vi "laplace_transform.vi"() -> ()   [LabVIEW 2020]
uses:
  <vilib>/Analysis/2dsp.llb/Real FFT.vi
  <vilib>/express/express analysis/Spectral/Block/exnSpectralBlock spectral measurements power poly.vi
  <vilib>/express/express analysis/Spectral/Block/exnSpectralBlock spectral measurements power WFM.vi
  <vilib>/express/express analysis/Spectral/Block/exnSpectralBlock spectral measurements power DDT.vi
  <vilib>/express/express analysis/Spectral/XNode/ExpressSpectralMeasurementsBlockNode.xnode
  <vilib>/Analysis/NI_AALPro.lvlib
  <vilib>/gmath/NI_Gmath.lvlib
panel:
  in  "end":dbl format="%.2f"
  out "Laplace Transform":dbl[](graph)
  out "Filtered Spectral Measurement":dynamicdata(graph)
  out "Spectral Measurement":cluster{"f0":dbl, "df":dbl, "magnitude":dbl[]}(graph)
  in  "shift?":bool
  in  "FFT size":i32=-1
  out "Fast Fourier Transform Graph":dbl[](graph)
  out "Amplitude vs Time (Chart)":waveform(dbl)(graph)
  out "Amplitude vs Time (Graph)":waveform(dbl)(graph)
  in  "path":path
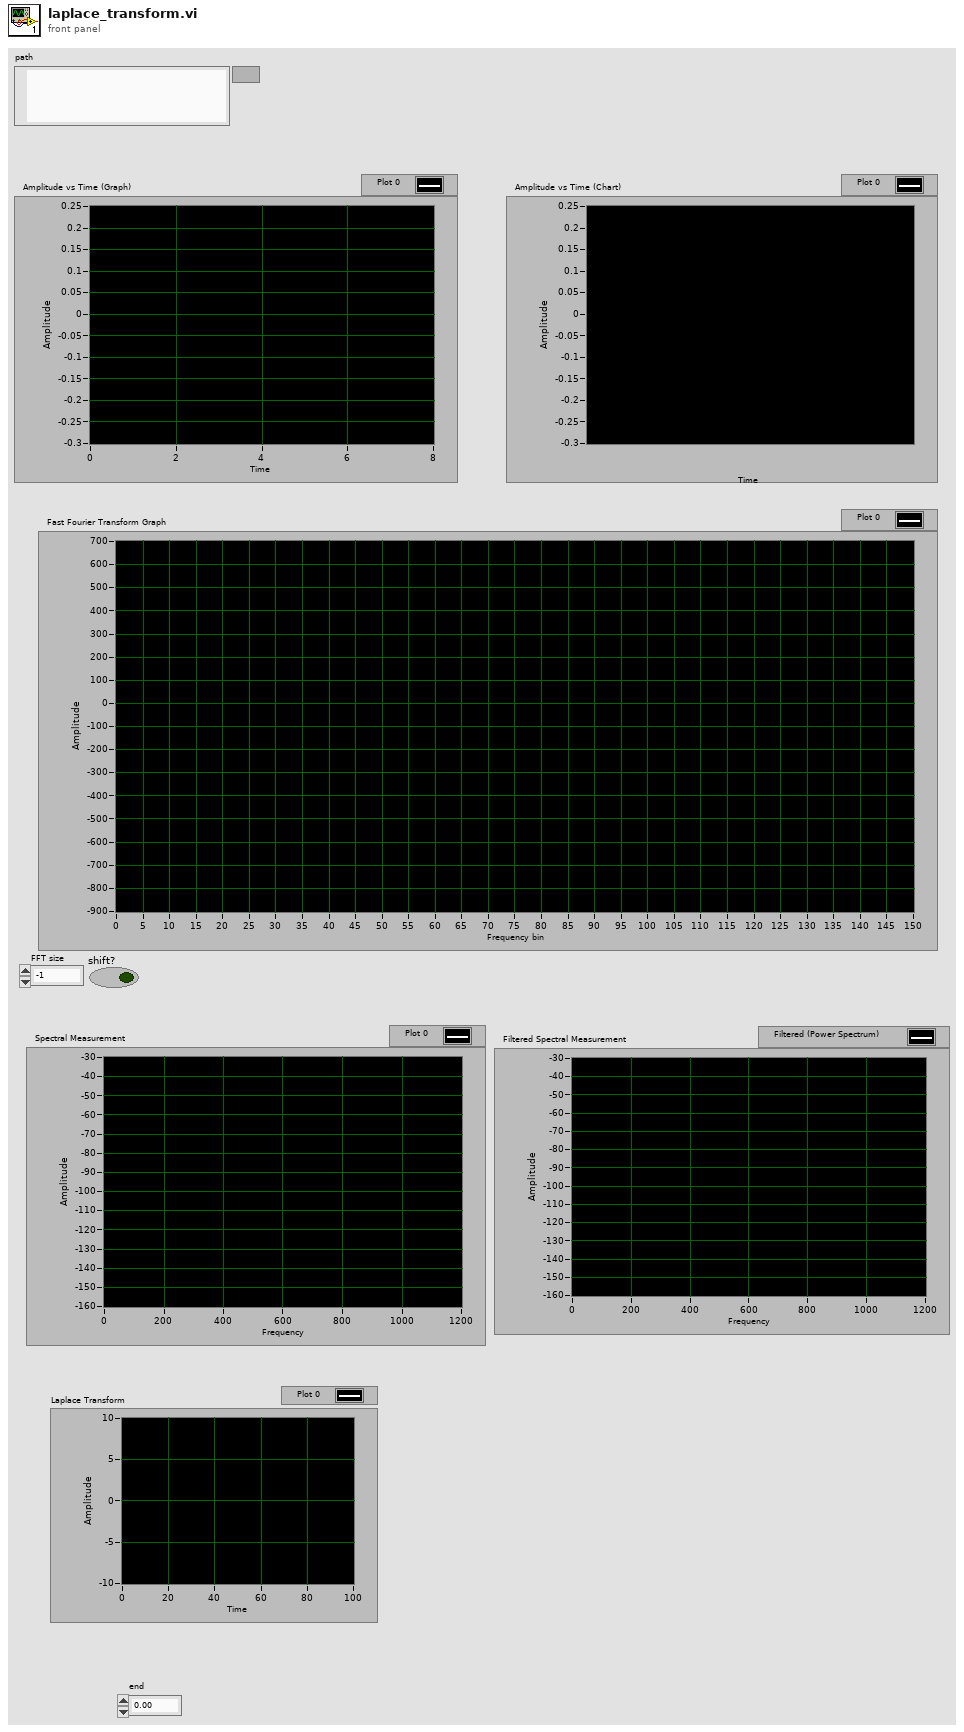
[diagram p1: front panel]
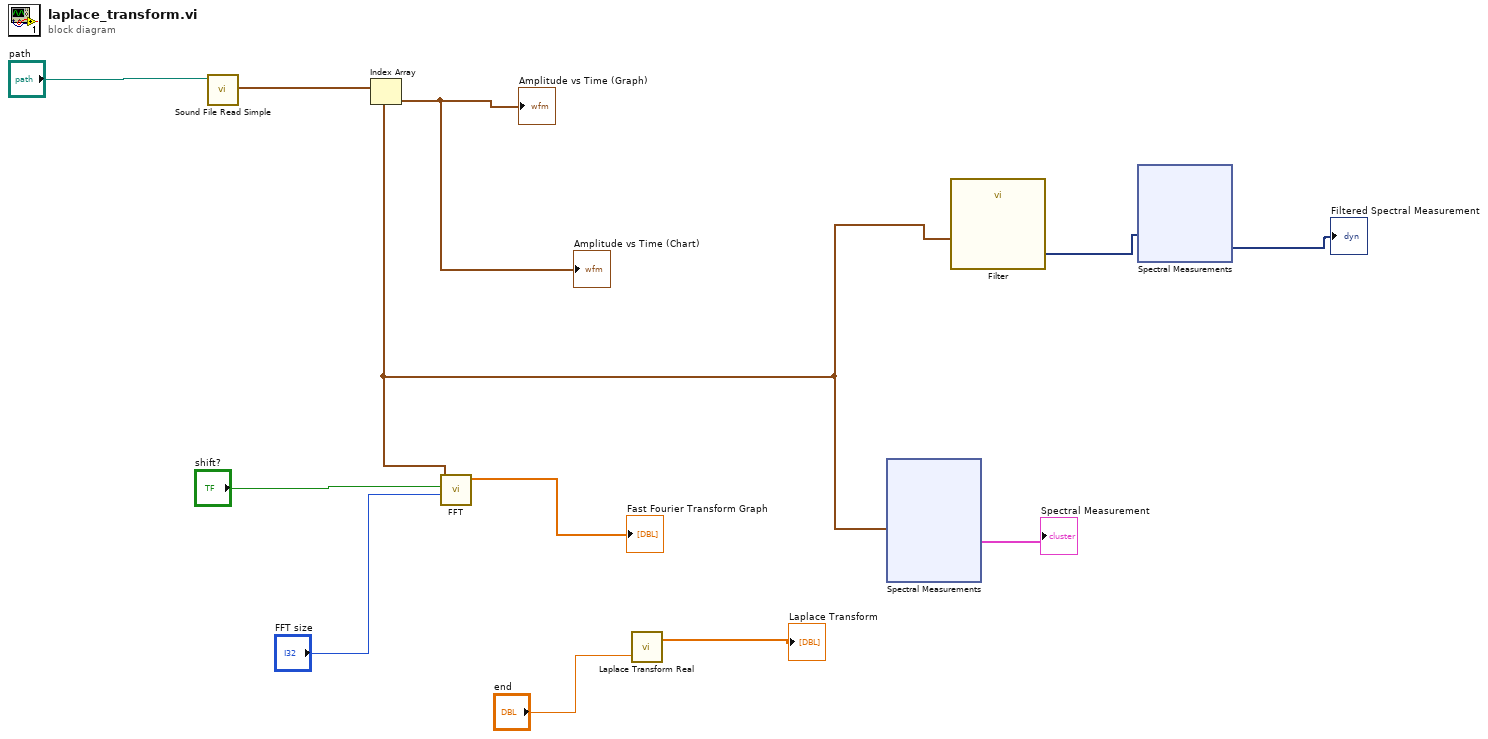
[diagram p0: block diagram]
diagram:
  n1 = call <vilib>:"Sound File Read Simple.vi"("path"="path") -> ("data"=w10:waveform(dbl)[])  [unwired: 7 in, 3 out]
  n2 = Index Array(array=w10) -> (element=w2:waveform(dbl))  [unwired: 1 in]
  "Amplitude vs Time (Graph)" <- w2
  "Amplitude vs Time (Chart)" <- w2
  n3 = call-poly <vilib>:"FFT.vi"("FFT size"="FFT size", "shift?"="shift?", "X"=w2) -> ("FFT {X}"=→"Fast Fourier Transform Graph":cdb[])  [unwired: 7 in, 1 out]
  n4 = call <vilib>:"Laplace Transform Real.vi"("end"="end") -> ("Laplace {X}"=→"Laplace Transform":dbl[])  [unwired: 1 in, 1 out]
  n5 = xnode "Spectral Measurements"("Signals"=w2) -> ("Power Spectrum"=→"Spectral Measurement":cluster{"f0":dbl, "df":dbl, "magnitude":dbl[]})  [unwired: 1 in, 1 out]
  n6 = call "Filter"("Signal"=w2) -> ("Filtered Signal"=w5:dynamicdata)  [unwired: 9 in, 1 out]
  n7 = xnode "Spectral Measurements"("Signals"=w5) -> ("Power Spectrum"=→"Filtered Spectral Measurement":dynamicdata)  [unwired: 1 in, 1 out]
